vi "Node HTTP Get.vi"(6 "Timeout ms (10000)":i32=10000, 7 "Node Name":string, 8 "error in (no error)":errorcluster, 10 "Path":string, 11 "VolatusAPI in":refnum<class "VolatusAPI.lvclass">) -> (0 "error out":errorcluster, 1 "Headers":string, 2 "Response":string, 3 "VolatusAPI out":refnum<class "VolatusAPI.lvclass">, 4 "Status Code":u32)   [LabVIEW 2020, in "Volatus.lvlib" / "VolatusAPI.lvclass"]
uses:
  VolatusAPI.lvclass
  VolatusAPI.lvclass/VolatusAPI.ctl
  <vilib>/httpClient/LabVIEWHTTPClient.lvlib
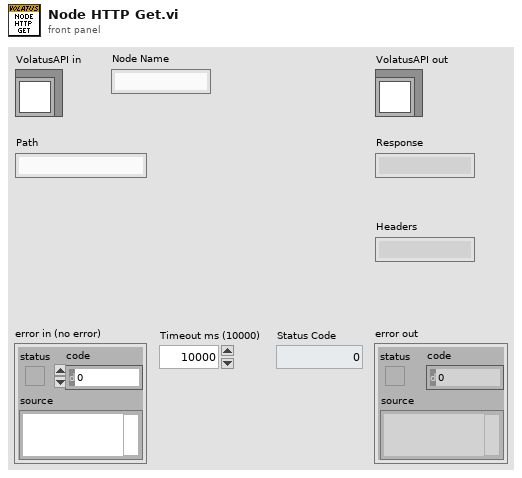
[diagram p1: front panel]
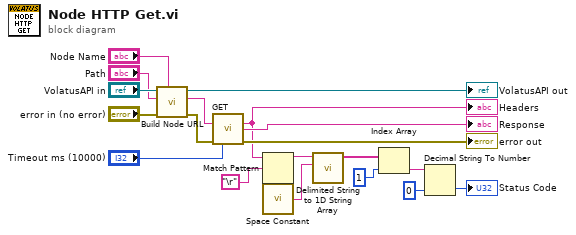
[diagram p0: block diagram]
diagram:
  n1 = call "Build Node URL.vi"("Node Name"="Node Name", "error in (no error)"="error in (no error)", "Path"="Path", "VolatusAPI in"="VolatusAPI in") -> ("error out"=w12:errorcluster, "Request URL"=w13:string, "VolatusAPI out"=→"VolatusAPI out":refnum<class "VolatusAPI.lvclass">)  [unwired: 5 in]
  n2 = call <vilib>:"GET.vi"("url"=w13, "error in (no error)"=w12, "timeout (10000)"="Timeout ms (10000)") -> ("headers"=w9:string, "body"=→"Response":string, "error out"=→"error out":errorcluster)  [unwired: 9 in, 1 out]
  "Headers" <- w9
  n3 = Match Pattern(string=w9, regular expression="\r") -> (before substring=w7:string)  [unwired: 1 in, 3 out]
  n4 = call <vilib>:"Space Constant.vi"() -> ("String"=w6:string)
  n5 = call <vilib>:"Delimited String to 1D String Array.vi"("delimiter"=w6, "delimited string"=w7) -> ("string array"=w5:string[])  [unwired: 9 in]
  n6 = Index Array(array=w5, index=1) -> (element=w3:string)
  n7 = Decimal String To Number(string=w3, default (0L)=u32 0 ("default (0 I32)")) -> (number=→"Status Code":u32)  [unwired: 1 in, 1 out]
